vi "GDSDialog_TwoButtonWindowsDialogLarge.vi"(1 "UserText":string, 2 "Button1Name":string, 3 "Button2Name":string, 4 "Cmd":refnum<user-event>, 5 "error in (no error)":errorcluster, 6 "DialogTitle":string, 7 "TimeOutTime(ms, ignored if not wired)":i32=-1, 8 "Icon":T1(ring)=enum."Information", 9 "Buttons_Font:Bold(False)":bool, 10 "Text.Justification(Left)":enum16{"Left", "Center", "Right"}(ring), 11 "OK_Font:Color(Black)":u32(colorbox)) -> (15 "Button1Pressed":bool=TRUE, 16 "TimeOut":bool, 19 "error out":errorcluster)   [LabVIEW 2020]
panel:
  in  "Button2":bool
  out "ShowIcon":T1(tab)
  out "Text":string
  in  "Button1":bool
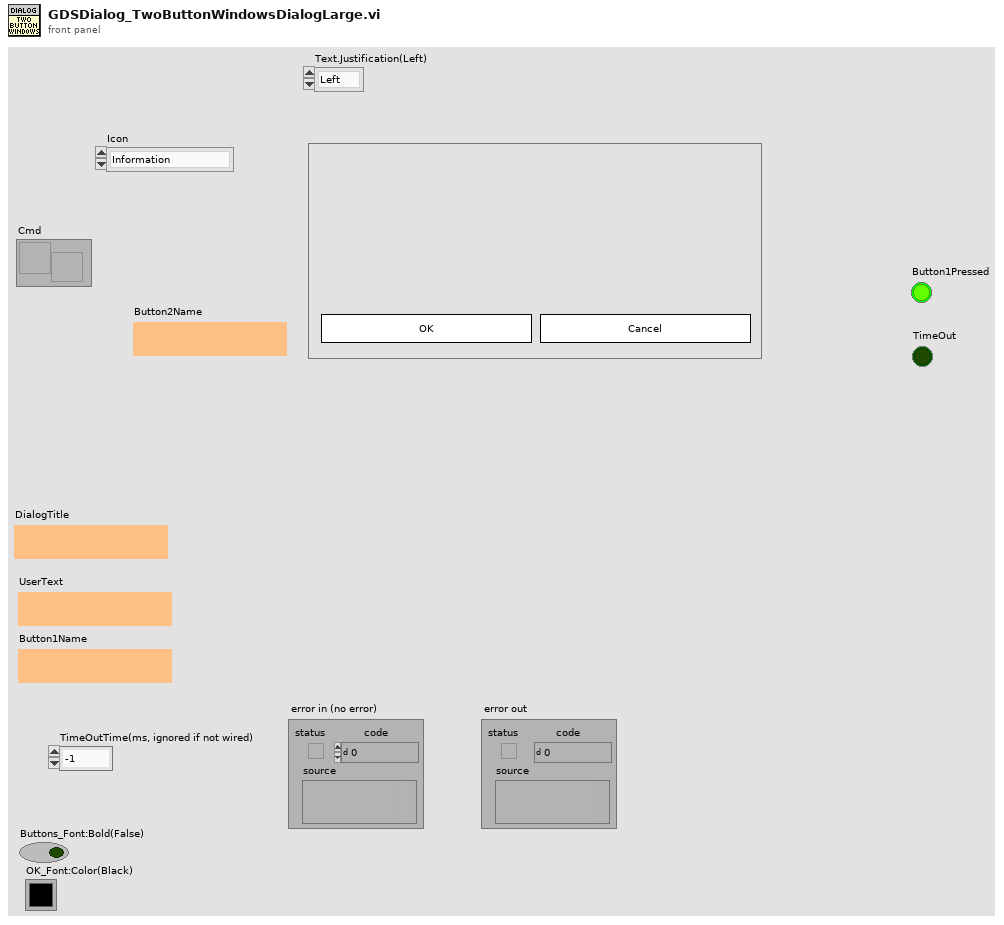
[diagram p1: front panel]
types:
  T1 = enum32{"None", "Stop", "Question", "Exclamation", "Information"}
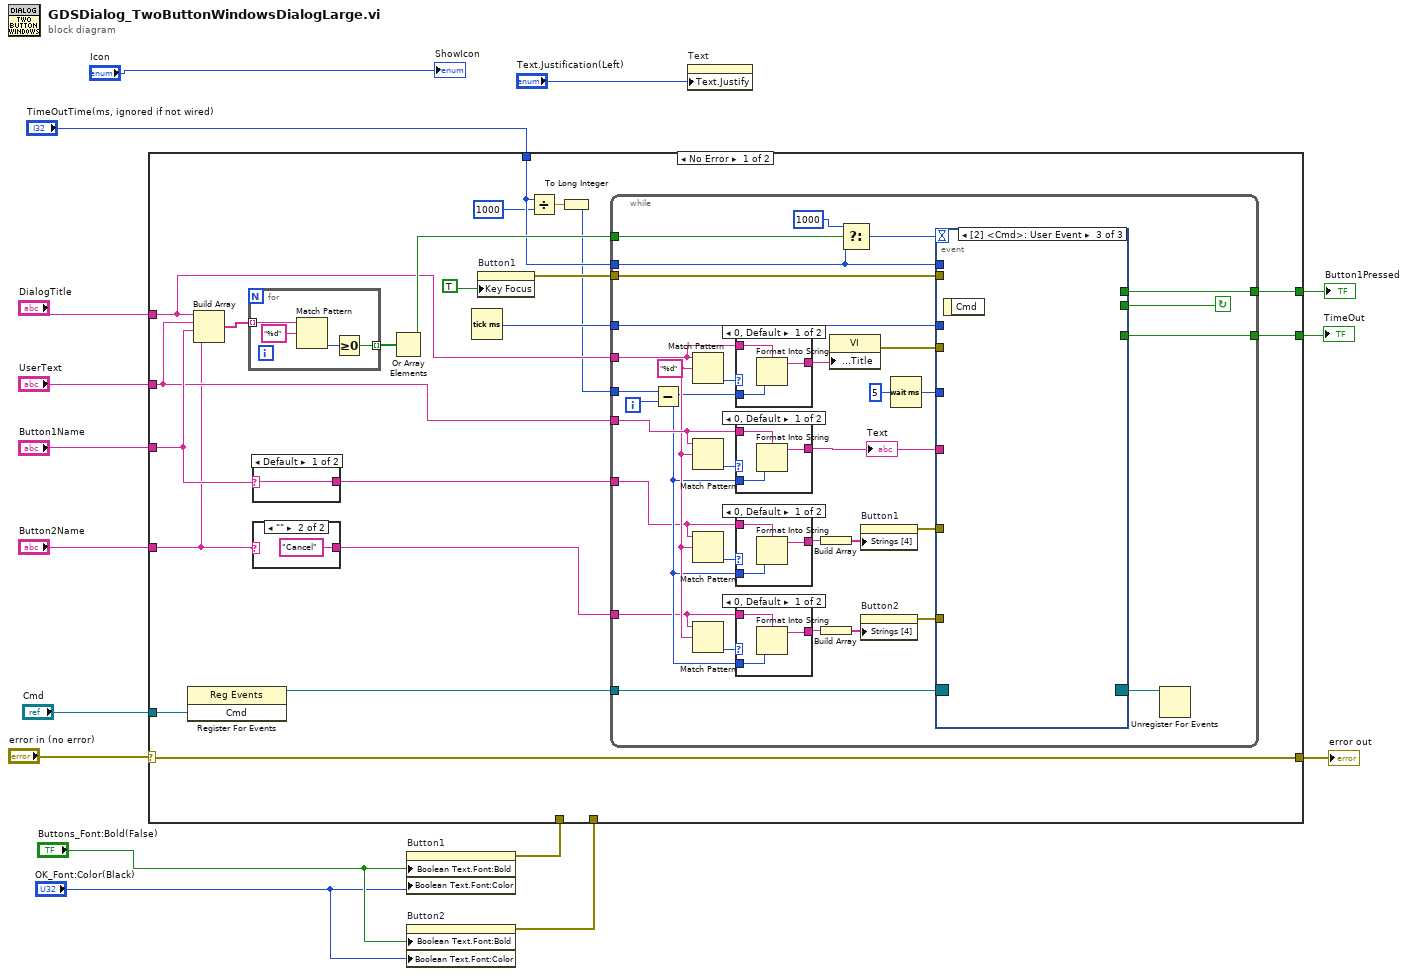
[diagram p0: block diagram]
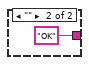
[diagram p3: hidden frame]
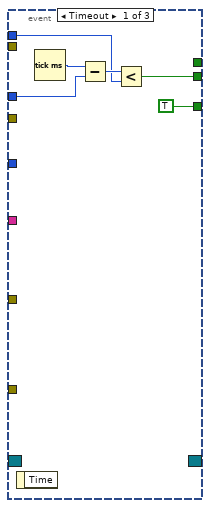
[diagram p8: hidden frame]
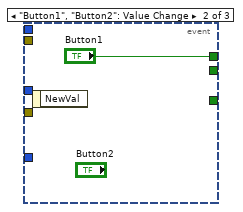
[diagram p9: hidden frame]
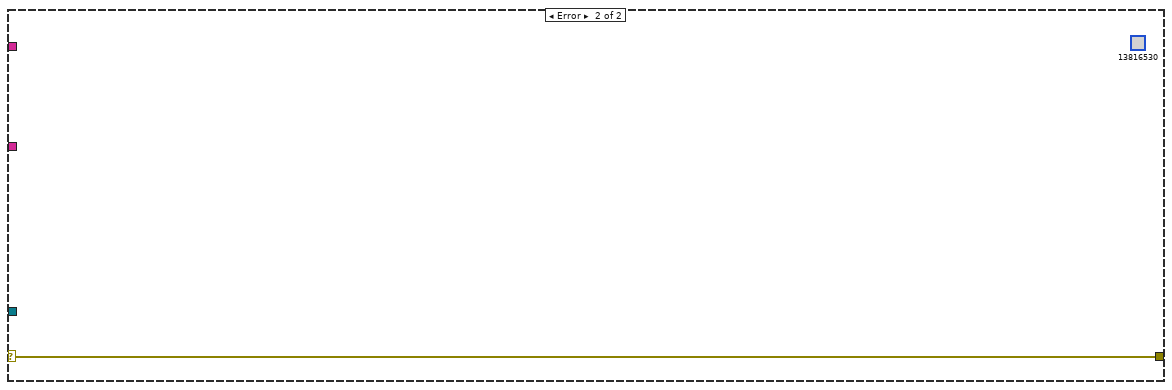
[diagram p10: hidden frame]
diagram:
  n1 = property on="Button1" class="Bool"("Boolean Text.Font:Bold"="Buttons_Font:Bold(False)", "Boolean Text.Font:Color"="OK_Font:Color(Black)") -> (error out=w7:errorcluster)  [unwired: 2 in, 1 out]
  n2 = property on="Button2" class="Bool"("Boolean Text.Font:Bold"="Buttons_Font:Bold(False)", "Boolean Text.Font:Color"="OK_Font:Color(Black)") -> (error out=w2:errorcluster)  [unwired: 2 in, 1 out]
  n3 = case shown="No Error" "error in (no error)" {
    selector: "error in (no error)" -> [w37 w103]
    tunnel: [w37 w103] -> w15
    tunnel: "UserText" -> [w23 _]
    tunnel: "DialogTitle" -> [w25 _]
    tunnel: "Button1Name" -> [w26 _]
    tunnel: "Cmd" -> [w34 _]
    tunnel: [w32 _] -> w10
    tunnel: "TimeOutTime(ms, ignored if not wired)" -> [w22 _]
    tunnel: [w31 _] -> w8
    tunnel: w7 -> [_ _]
    tunnel: w2 -> [_ _]
    tunnel: "Button2Name" -> [w18 _]
    frame No Error {
      n4 = register-events(w34) -> (reference out=w33:refnum<event-registration>)  [unwired: 2 in, 1 out]
      n5 = Build Array(w25, w23, w26, w18) -> (w30:string[])
      n6 = for {
        tunnel: w30 -> [w102] mode=indexing
        tunnel: [w99] -> w28 mode=indexing
        n7 = Match Pattern(string=w102, regular expression="%d") -> (offset past match=w100:i32)  [unwired: 1 in, 3 out]
        n8 = Greater Or Equal To 0?(x=w100) -> (x >= 0?=w99:bool)
      }
      n9 = case shown="Default" w26 {
        selector: w26 -> [w40 _]
        tunnel: [w40 "OK"] -> w24
        frame Default {
        }
        frame "" {
        }
      }
      n10 = case shown="\"\"" w18 {
        selector: w18 -> [w38 _]
        tunnel: [w38 "Cancel"] -> w17
        frame Default {
        }
        frame "" {
        }
      }
      n11 = Or Array Elements(Boolean array=w28) -> (logical OR=w27:bool)
      n12 = Tick Count (ms)() -> (millisecond timer value=w29:u32)
      n13 = property on="Button1" class="Bool"("Key Focus"=TRUE) -> (error out=w35:errorcluster)  [unwired: 2 in, 1 out]
      n14 = Divide(x=w22, y=1000) -> (x/y=w20:dbl)
      n15 = To Long Integer(number=w20) -> (32bit integer=w19:i32)
      n16 = while {
        tunnel: w35 -> [w75]
        tunnel: w33 -> [w74]
        tunnel: [w72] -> w32
        tunnel: w22 -> [w67]
        tunnel: [w71] -> w31
        tunnel: w29 -> [w70]
        tunnel: w27 -> [w68]
        tunnel: w25 -> [w61]
        tunnel: w23 -> [w55]
        tunnel: w24 -> [w49]
        tunnel: w19 -> [w60]
        tunnel: w17 -> [w48]
        i -> [w59]
        stop <- w69 continue-if-true
        w51 = "%d" ("regular expression")
        n17 = Subtract(x=w60, y=w59) -> (x-y=w50:i32)
        n18 = Match Pattern(string=w61, regular expression=w51) -> (offset past match=w63:i32)  [unwired: 1 in, 3 out]
        n19 = Match Pattern(string=w55, regular expression=w51) -> (offset past match=w58:i32)  [unwired: 1 in, 3 out]
        n20 = Match Pattern(string=w49, regular expression=w51) -> (offset past match=w57:i32)  [unwired: 1 in, 3 out]
        n21 = Match Pattern(string=w48, regular expression=w51) -> (offset past match=w53:i32)  [unwired: 1 in, 3 out]
        n22 = case shown="0, Default" w63 {
          tunnel: [w88 w91] -> w62
          tunnel: w61 -> [w90 w91]
          tunnel: w50 -> [w89 _]
          frame 0, Default {
            n23 = Format Into String(format string=w90, w89) -> (resulting string=w88:string)  [unwired: 2 in, 1 out]
          }
          frame -1 {
          }
        }
        n24 = case shown="0, Default" w58 {
          tunnel: [w84 w87] -> w44
          tunnel: w55 -> [w86 w87]
          tunnel: w50 -> [w85 _]
          frame 0, Default {
            n25 = Format Into String(format string=w86, w85) -> (resulting string=w84:string)  [unwired: 2 in, 1 out]
          }
          frame -1 {
          }
        }
        "Text" <- w44
        n26 = case shown="0, Default" w57 {
          tunnel: [w80 w83] -> w56
          tunnel: w49 -> [w82 w83]
          tunnel: w50 -> [w81 _]
          frame 0, Default {
            n27 = Format Into String(format string=w82, w81) -> (resulting string=w80:string)  [unwired: 2 in, 1 out]
          }
          frame -1 {
          }
        }
        n28 = case shown="0, Default" w53 {
          tunnel: [w76 w79] -> w54
          tunnel: w48 -> [w78 w79]
          tunnel: w50 -> [w77 _]
          frame 0, Default {
            n29 = Format Into String(format string=w78, w77) -> (resulting string=w76:string)  [unwired: 2 in, 1 out]
          }
          frame -1 {
          }
        }
        n30 = Build Array(w56) -> (w64:string[])
        n31 = Build Array(w54) -> (w52:string[])
        n32 = property class="VI"("Front Panel Window:Title"=w62) -> (error out=w45:errorcluster)  [unwired: 2 in, 1 out]
        n33 = Select(t=1000, s=w68, f=w67) -> (s? t:f=w66:i32)
        n34 = property on="Button1" class="Bool"("Strings [4]"=w64) -> (error out=w43:errorcluster)  [unwired: 2 in, 1 out]
        n35 = property on="Button2" class="Bool"("Strings [4]"=w52) -> (error out=w42:errorcluster)  [unwired: 2 in, 1 out]
        n36 = Wait (ms)(milliseconds to wait=u32 5) -> (millisecond timer value=w46:u32)
        n37 = event shown="[2] <Cmd>: User Event" {
          selector: w74 -> [_ _ _]
          dyn-events: [_ _ _] -> w73
          timeout: w66 -> [_ _ _]
          tunnel: w75 -> [_ _ _]
          tunnel: [_ "Button1" _] -> w72
          tunnel: [TRUE _ _] -> w71
          tunnel: w70 -> [w95 _ _]
          tunnel: [w93 _ _] -> w69
          tunnel: w67 -> [w92 _ _]
          tunnel: w46 -> [_ _ _]
          tunnel: w45 -> [_ _ _]
          tunnel: w44 -> [_ _ _]
          tunnel: w43 -> [_ _ _]
          tunnel: w42 -> [_ _ _]
          event Timeout {
            n38 = event-data() -> ()  [unwired: 1 in, 1 out]
            n39 = Tick Count (ms)() -> (millisecond timer value=w96:u32)
            n40 = Subtract(x=w96, y=w95) -> (x-y=w94:u32)
            n41 = Less?(x=w94, y=w92) -> (x < y?=w93:bool)
          }
          event "Button1", "Button2": Value Change {
            n42 = event-data() -> ()  [unwired: 1 in, 1 out]
          }
          event User Event {
            n43 = event-data() -> ()  [unwired: 1 in, 1 out]
          }
        }
        n44 = Unregister For Events(event registration refnum=w73) -> ()  [unwired: 1 in, 1 out]
      }
    }
    frame Error {
      (unwired) u32 13816530 ("BgColor")
    }
  }
  "error out" <- w15
  "Button1Pressed" <- w10
  "TimeOut" <- w8
  n45 = property on="Text" class="Str"("Text.Justify"="Text.Justification(Left)") -> ()  [unwired: 2 in, 2 out]
  "ShowIcon" <- "Icon"
